vi "Drive control.vi"(8 "Right stick X":dbl, 9 "Left stick Y":dbl, 10 "Left stick X":dbl, 11 "Gyro angle":dbl) -> (1 "Rotation":dbl, 2 "Direction":dbl, 3 "Magnitude":dbl)   [LabVIEW 2014]
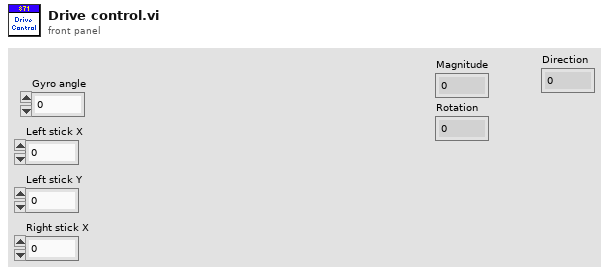
[diagram p1: front panel]
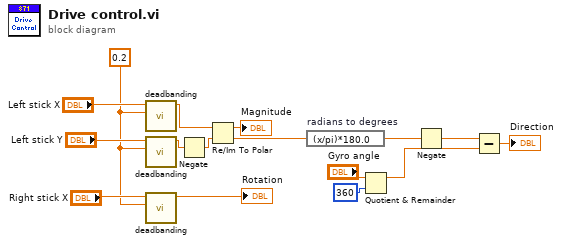
[diagram p0: block diagram]
diagram:
  w1 = 0.2
  n1 = call "deadbanding.vi"("width"=w1, "joystick"="Left stick X") -> ("deadbanded"=w4:dbl)  [unwired: 9 in]
  n2 = call "deadbanding.vi"("width"=w1, "joystick"="Left stick Y") -> ("deadbanded"=w2:dbl)  [unwired: 9 in]
  n3 = call "deadbanding.vi"("width"=w1, "joystick"="Right stick X") -> ("deadbanded"=→"Rotation":dbl)  [unwired: 9 in]
  n4 = Negate(x=w2) -> (-x=w3:dbl)
  n5 = Re/Im To Polar(2:w3, 3:w4) -> (0:w11:dbl, 1:→"Magnitude":dbl)
  n6 = expression code="(x/pi)*180.0" "radians to degrees"(w11) -> (w5:dbl)
  n7 = Quotient & Remainder(x="Gyro angle", y=360) -> (x-y*floor(x/y)=w13:dbl)  [unwired: 1 out]
  n8 = Negate(x=w5) -> (-x=w6:dbl)
  n9 = Subtract(x=w6, y=w13) -> (x-y=→"Direction":dbl)
